vi "Calculate field raster.vi"(0 "# Fields across x":i8, 1 "# Fields across y":i8, 2 "Index (0 to n-1)":i32) -> (3 "y":dbl, 5 "x":dbl, 6 "dx":dbl, 7 "dy":dbl, 8 "k":dbl, 9 "j":dbl)   [LabVIEW 2016]
uses:
  new-h-nu-ixon/stage globals.vi
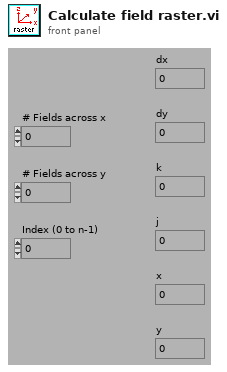
[diagram p1: front panel]
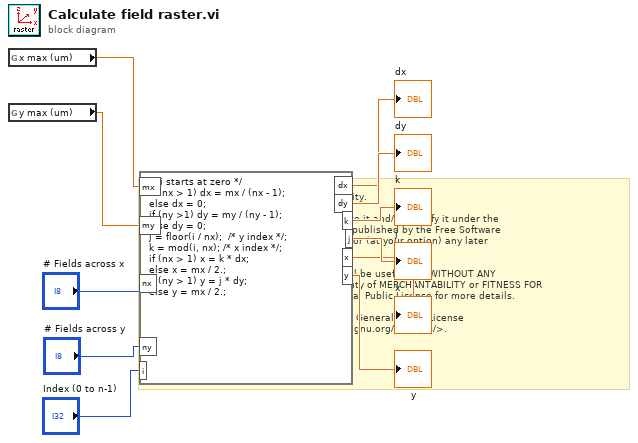
[diagram p0: block diagram]
diagram:
  # "This file is part of Glimpse. \nCopyright 2014 Jeff Gelles, Brandeis University.    \n\nGlimpse is free software: you can redistribute it and/or modify it under the \nterms of the GNU General Public License as published by the Free Software \nFoundation, either version 3 of the License, or (at your option) any later \nversion.\n\nGlimpse is distributed in the hope that it will be useful, but WITHOUT ANY \nWARRANTY; without even the implied warranty of MERCHANTABILITY or FITNESS FOR \nA PARTICULAR PURPOSE.  See the GNU General Public License for more details.\n\nYou should have received a copy of the GNU General Public License\nalong with Glimpse.  If not, see <http://www.gnu.org/licenses/>."
  n1 = global read "stage globals.vi" "x max (um)"() -> (w2:ext)
  n2 = global read "stage globals.vi" "y max (um)"() -> (w1:ext)
  n3 = formula code="/* i starts at zero */\nif (nx > 1) dx = mx / (nx - 1);\nelse dx = 0;\nif (ny >1) dy = my / (ny - 1);\nelse dy = 0;\nj = floor(i / nx);  /* y index */;\nk = mod(i, nx); /* x index */;\nif (nx > 1) x = k * dx;\nelse x = mx / 2.;\nif (ny > 1) y = j * dy;\nelse y = mx / 2.;"("nx"="# Fields across x", "ny"="# Fields across y", "mx"=w2, "i"="Index (0 to n-1)", "my"=w1) -> ("dx"=→"dx":dbl, "dy"=→"dy":dbl, "k"=→"k":dbl, "j"=→"j":dbl, "x"=→"x":dbl, "y"=→"y":dbl)
